vi "Simulation.vi"(8 "error in (no error)":errorcluster, 11 "MB Sim Base in":refnum<class "iC7-INU.lvclass">) -> (0 "error out":errorcluster)   [LabVIEW 2021, in "iC7-INU.lvclass"]
uses:
  iC7-INU.lvclass
  C:/S2L_Dev/LV2021/lv-Vessel_Simulator/MB Slave Simulator Base/MB Slave Simulator Base.lvclass
  C:/Program Files (x86)/National Instruments/LabVIEW 2021/user.lib/S2 Labs/Module Framework/Modules/Modbus/Modbus Slave Base/Modbus Slave Base.lvclass
  MB Slave Simulator Base/MB Slave Simulator Base.lvclass/MB Slave Simulator Base.ctl
  <userlib>/S2 Labs/Module Framework/Modules/Modbus/Modbus Slave Base/Modbus Slave Base.lvclass/Modbus Slave Base.ctl
  MB Slave Simulator Base/Accessors/Read Initialized.vi
  <userlib>/S2 Labs/Module Framework/Modules/Modbus/Modbus Slave Base/Read MB Ref.vi
  <userlib>/S2 Labs/Modbus Toolkit/Slave/S2L Modbus Slave.lvclass
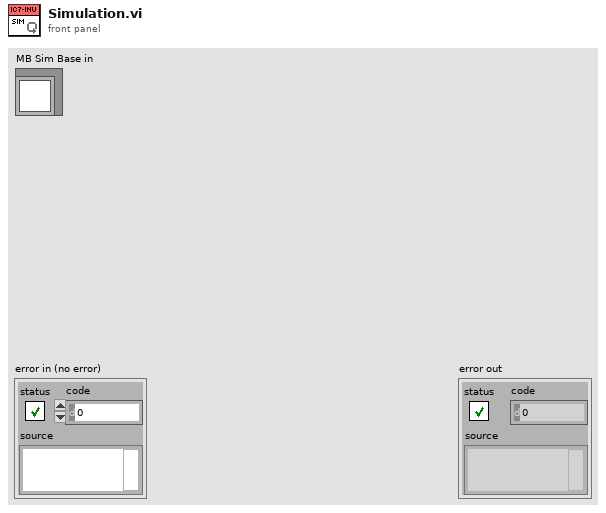
[diagram p1: front panel]
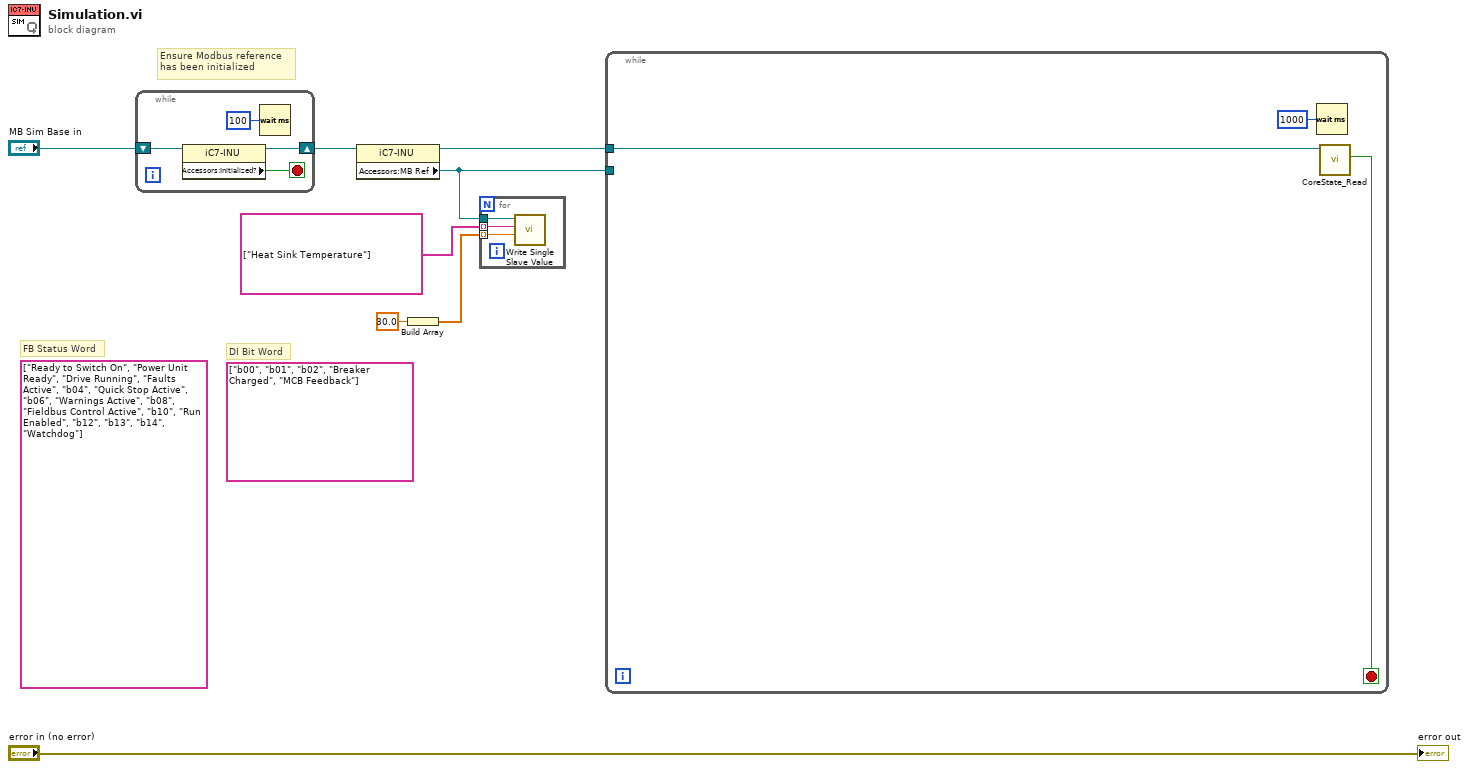
[diagram p0: block diagram]
diagram:
  (unwired) string[] ["b00", "b01", "b02", "Breaker Charged", "MCB Feedback"] ("LUT")
  (unwired) string[] ["Ready to Switch On", "Power Unit Ready", "Drive Running", "Faults Active", "b04", "Quick Stop Active", "b06", "Warnings Active", "b08", "Fieldbus Control Active", "b10", "Run Enabled", "b12", "b13", "b14", "Watchdog"] ("LUT")
  # "DI Bit Word"
  # "FB Status Word"
  # "Ensure Modbus reference\nhas been initialized"
  n1 = while {
    shift-right: [w10] -> w6
    shift-left: "MB Sim Base in" -> [w11]
    stop <- w9 stop-if-true
    n2 = property class="iC7-INU"(reference=w11) -> (reference out=w10:refnum<class "iC7-INU.lvclass">, "Accessors:Initialized?"=w9:bool)  [unwired: 1 in, 1 out]
    n3 = Wait (ms)(milliseconds to wait=u32 100) -> ()  [unwired: 1 out]
  }
  n4 = property class="iC7-INU"(reference=w6) -> (reference out=w5:refnum<class "iC7-INU.lvclass">, "Accessors:MB Ref"=w4:refnum<class "S2L Modbus Slave.lvclass">)  [unwired: 1 in, 1 out]
  n5 = Build Array(30.0 ("element")) -> (w8:dbl[])
  n6 = for {
    tunnel: w4 -> [w15]
    tunnel: string[] ["Heat Sink Temperature"] ("Label") -> [w14] mode=indexing
    tunnel: w8 -> [w13] mode=indexing
    n7 = call-dynamic "Write Single Slave Value.vi"("Value"=w13, "Label"=w14, "S2L Modbus Slave in"=w15) -> ()  [unwired: 7 in, 2 out]
  }
  n8 = while {
    tunnel: w5 -> [w17]
    tunnel: w4 -> [_]
    stop <- w16 stop-if-true
    n9 = Wait (ms)(milliseconds to wait=u32 1000) -> ()  [unwired: 1 out]
    n10 = call-dynamic "CoreState_Read.vi"("Module in"=w17) -> ("Stopped?"=w16:bool)  [unwired: 8 in, 2 out]
  }
  "error out" <- "error in (no error)"
